vi "Set Detection.vi"(8 "error in (no error)":errorcluster, 9 "Optical Path":T1=1 items=["Eyepieces"=1, "Right"=2, "Bottom"=3, "Left"=4], 10 "Filter Position":T2=1 items=["1"=1, "2"=2, "3"=3, "4"=4, "5"=5, "6"=6], 11 "Ti2 in":refnum<class "Microscope.lvclass">) -> (0 "error out":errorcluster, 3 "Ti2 out":refnum<class "Microscope.lvclass">)   [LabVIEW 2023, in "Microscope.lvlib" / "Microscope.lvclass"]
uses:
  Microscope.lvclass
  ti2lv/ti2_filterPos.ctl
  ti2lv/ti2_lightPath.ctl
  Microscope.lvclass/Microscope.ctl
  ti2lv/ti2lv.lvlib
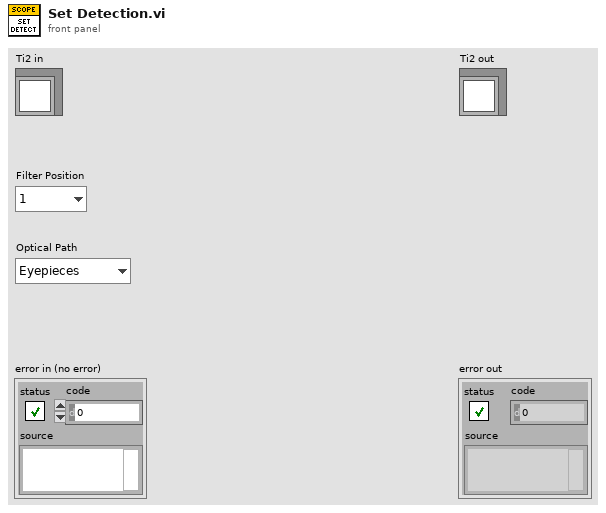
[diagram p1: front panel]
types:
  T1 = typedef "ti2lv.lvlib/ti2_lightPath.ctl" = i32
  T2 = typedef "ti2lv.lvlib/ti2_filterPos.ctl" = u16
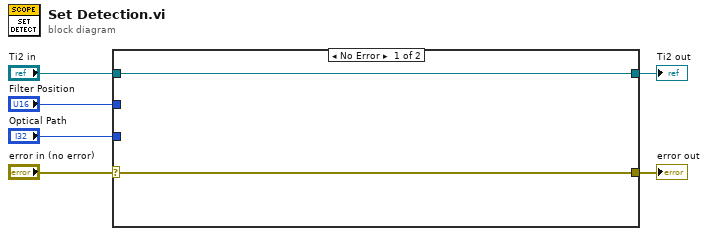
[diagram p0: block diagram]
diagram:
  n1 = case shown="No Error" "error in (no error)" {
    selector: "error in (no error)" -> [w7 w10]
    tunnel: [w7 w10] -> w5
    tunnel: [w8 w9] -> w3
    tunnel: "Ti2 in" -> [w8 w9]
    tunnel: "Optical Path" -> [_ _]
    tunnel: "Filter Position" -> [_ _]
    frame No Error {
    }
    frame Error {
    }
  }
  "error out" <- w5
  "Ti2 out" <- w3
